vi "Send Param Helper.vi"(8 "error in (no error)":errorcluster, 9 "Parameter":refnum<class "Value.lvclass">, 10 "Param Class":string, 11 "Param Event":refnum<user-event>) -> (0 "error out":errorcluster)   [LabVIEW 2020]
uses:
  Error Result/Error Result.lvclass
  Value/Value.lvclass
  C:/dev/lv/2020/lv-promises/Promises/Value/Value.lvclass
  C:/dev/lv/2020/lv-promises/Promises/Error Result/Error Result.lvclass
  Parameter Data.ctl
  Promises.lvlib
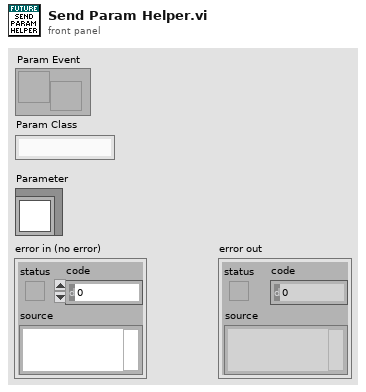
[diagram p1: front panel]
types:
  T1 = cluster{"Parameter":refnum<class "Value.lvclass">}
  T2 = cluster{"Error Result out":refnum<class "Error Result.lvclass">}
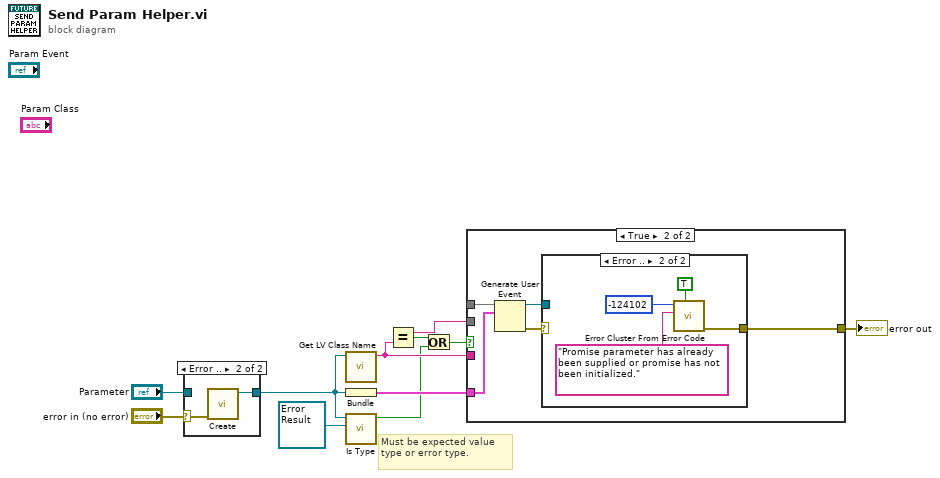
[diagram p0: block diagram]
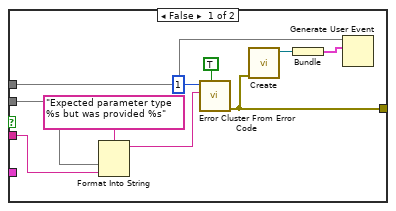
[diagram p3: hidden frame]
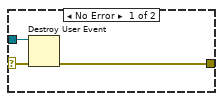
[diagram p4: hidden frame]
diagram:
  # "Must be expected value type or error type."
  n1 = case shown="Error .." "error in (no error)" {
    selector: "error in (no error)" -> [_ w14]
    tunnel: "Parameter" -> [w12 _]
    tunnel: [w12 w13] -> w1
    frame No Error {
    }
    frame Error {
      n2 = call "Create.vi"("error in (no error)"=w14) -> ("Error Result out"=w13:refnum<class "Error Result.lvclass">)  [unwired: 9 in, 1 out]
    }
  }
  n3 = call <vilib>:"Get LV Class Name.vi"("object"=w1) -> ("class name"=w9:string)  [unwired: 9 in, 1 out]
  n4 = Bundle("Parameter"=w1) -> (w7:T1)  [unwired: 1 in]
  n5 = call "Is Type.vi"("Type"=refnum<class "Error Result.lvclass"> refnum ("Futures:Error Result.lvclass"), "Value"=w1) -> ("Type Matches"=w4:bool)  [unwired: 9 in]
  n6 = Equal?(y=w9) -> (x=w11:string, x = y?=w10:bool)
  n7 = Or(x=w10, y=w4) -> (x .or. y?=w5:bool)
  n8 = case shown="True" w5 {
    tunnel: w7 -> [_ w25]
    tunnel: w11 -> [w24 _]
    tunnel: w9 -> [w23 _]
    tunnel: _ -> [w17 w29]
    tunnel: [w18 w26] -> w8
    frame False {
      n9 = Format Into String(format string="Expected parameter type %s but was provided %s", w24, w23) -> (resulting string=w20:string)  [unwired: 2 in, 1 out]
      n10 = call <vilib>:"Error Cluster From Error Code.vi"("show call chain? (False)"=TRUE, "error message (\"\")"=w20, "error code (0)"=1) -> ("error out"=w18:errorcluster)  [unwired: 6 in]
      n11 = call "Create.vi"("error in (no error)"=w18) -> ("Error Result out"=w16:refnum<class "Error Result.lvclass">)  [unwired: 9 in, 1 out]
      n12 = Bundle("Error Result out"=w16) -> (w15:T2)  [unwired: 1 in]
      n13 = Generate User Event(user event=w17, event data cluster=w15) -> ()  [unwired: 2 in, 2 out]
    }
    frame True {
      n14 = Generate User Event(user event=w29, event data cluster=w25) -> (user event out=w27:refnum<user-event>, error out=w28:errorcluster)  [unwired: 2 in]
      n15 = case shown="Error .." w28 {
        selector: w28 -> [w31 _]
        tunnel: w27 -> [w32 _]
        tunnel: [w30 w36] -> w26
        frame No Error {
          n16 = Destroy User Event(user event=w32, error in=w31) -> (error out=w30:errorcluster)
        }
        frame Error {
          n17 = call <vilib>:"Error Cluster From Error Code.vi"("show call chain? (False)"=TRUE, "error message (\"\")"="Promise parameter has already been supplied or promise has not been initialized.", "error code (0)"=-124102) -> ("error out"=w36:errorcluster)  [unwired: 6 in]
        }
      }
    }
  }
  "error out" <- w8
